vi "draw.vi"(8 "error in (no error)":errorcluster, 11 "afSquare in":refnum<class "afSquare.lvclass">) -> (0 "error out":errorcluster, 3 "afSquare out":refnum<class "afSquare.lvclass">)   [LabVIEW 2018, in "afSquare.lvclass"]
uses:
  afSquare.lvclass
  ConsoleOut/Print Options.ctl
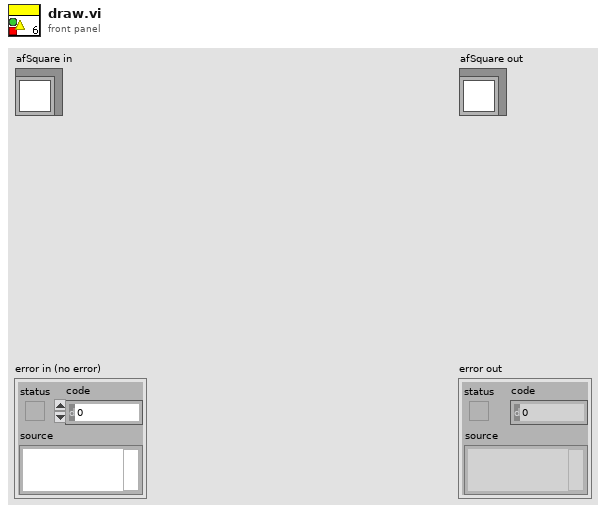
[diagram p1: front panel]
types:
  T1 = typedef "Print Options.ctl" = enum16{"Create", "Get Reference", "Print", "Print Header", "Close"}
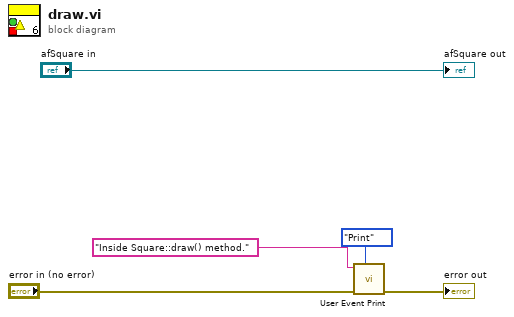
[diagram p0: block diagram]
diagram:
  n1 = call "User Event Print.vi"("Options"=Print_Options."Print", "error in (no error)"="error in (no error)", "String to Print"="Inside Square::draw() method." ("message")) -> ("error out"=→"error out":errorcluster)  [unwired: 7 in, 1 out]
  "afSquare out" <- "afSquare in"
